vi "Linear_voltage_converter.vi"(1 "Caib const A,B":dbl[](array[numeric]) format="%.4f", 2 "Voltage array":dbl[](array[numeric]) format="%.2f") -> (0 "Converted array":dbl[](array[numeric]) format="%.2f")   [LabVIEW 2010]
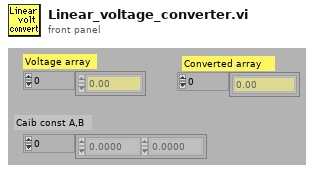
[diagram p1: front panel]
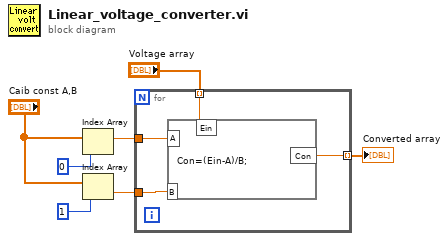
[diagram p0: block diagram]
diagram:
  n1 = Index Array(array="Caib const A,B", index=0) -> (element=w4:dbl)
  n2 = Index Array(array="Caib const A,B", index=1) -> (element=w3:dbl)
  n3 = for {
    tunnel: w4 -> [w11]
    tunnel: w3 -> [w10]
    tunnel: "Voltage array" -> [w9] mode=indexing
    tunnel: [w8] -> w1 mode=indexing
    n4 = formula code="Con=(Ein-A)/B;"("Ein"=w9, "B"=w10, "A"=w11) -> ("Con"=w8:dbl)
  }
  "Converted array" <- w1
